vi "Initialize.vi"(8 "error in (no error)":errorcluster, 10 "Instrument Refnum in":refnum<visa-resource-name>, 11 "PCI-4070 in":refnum<class "PCI-4070.lvclass">) -> (0 "error out":errorcluster, 2 "Result Text":string="PCI-4070 has been initialized", 3 "PCI-4070 out":refnum<class "PCI-4070.lvclass">)   [LabVIEW 2012, in "PCI-4070.lvclass"]
uses:
  PCI-4070.lvclass
  DMM Base/DMM.lvclass
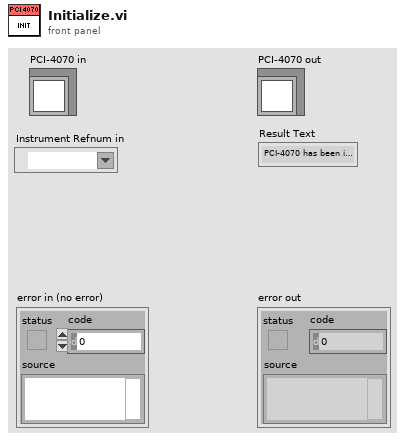
[diagram p1: front panel]
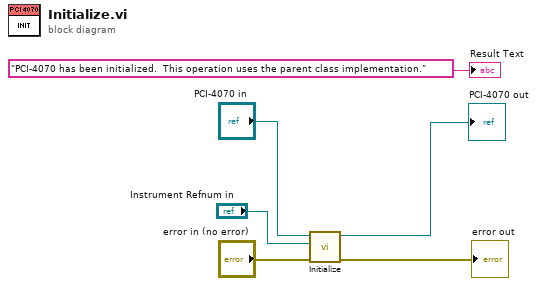
[diagram p0: block diagram]
diagram:
  n1 = call-parent "Initialize.vi"("error in (no error)"="error in (no error)", "Instrument Refnum in"="Instrument Refnum in", "DMM in"="PCI-4070 in") -> ("error out"=→"error out":errorcluster, "DMM out"=→"PCI-4070 out":refnum<class "PCI-4070.lvclass">)  [unwired: 6 in, 1 out]
  "Result Text" <- "PCI-4070 has been initialized.  This operation uses the parent class implementation." ("message")
